vi "GetMTSUMData.vi"(10 "RCNO":string="A150100736") -> (0 "bin4":i32, 1 "bin3":i32, 2 "bin2":i32, 3 "bin1":i32, 4 "Program":string, 5 "input":i32, 6 "EndDate":string, 7 "StartDate":string, 8 "Yield":dbl)   [LabVIEW 2012]
uses:
  <vilib>/addons/database/Auxilliary.llb/DB Tools Cursor Type.ctl
  <vilib>/addons/database/Connection.llb/DB Tools Open Connec (Path).vi
  <vilib>/addons/database/Connection.llb/Conn Execute.vi
  <vilib>/addons/database/Recordset.llb/Rec Fetch String Data (R).vi
  <vilib>/addons/database/Recordset.llb/Rec Fetch Integer Data (R).vi
  <vilib>/addons/database/Recordset.llb/Rec Destroy - Connection.vi
  <vilib>/addons/database/NI_Database_API.lvlib
panel:
  out "error out":errorcluster
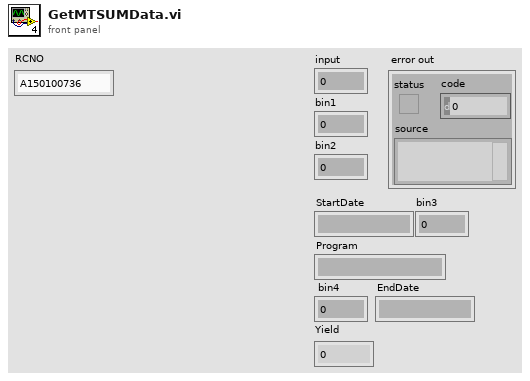
[diagram p1: front panel]
types:
  T1 = typedef "NI_Database_API.lvlib/DB Tools Cursor Type.ctl" = enum16{"forward-only", "keyset", "dynamic", "static"}
  T2 = typedef "NI_Database_API.lvlib/Conn ObjectReference.ctl" = refnum<k1>
  T3 = typedef "NI_Database_API.lvlib/Rec ObjectReference.ctl" = refnum<k1>
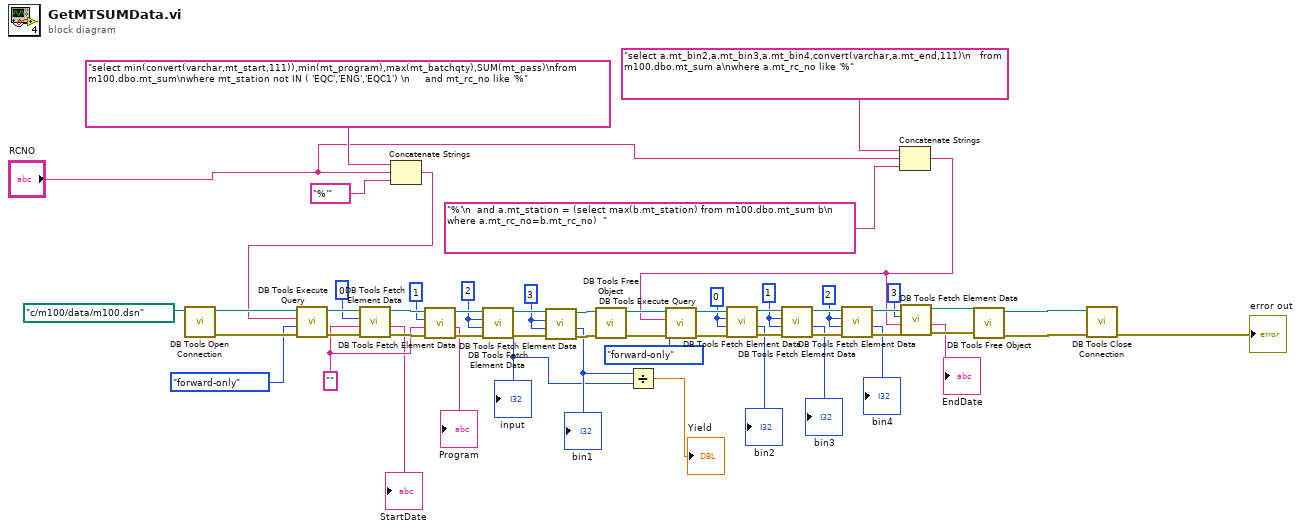
[diagram p0: block diagram]
diagram:
  w23 = 2
  w24 = 1
  w25 = 0
  w38 = 3
  w39 = 2
  w42 = ""
  n1 = call-poly <vilib>:"DB Tools Open Connection.vi"("connection information"=path "c:/m100/data/m100.dsn") -> ("error out"=w52:errorcluster, "connection reference"=w54:T2)  [unwired: 7 in]
  n2 = Concatenate Strings("select min(convert(varchar,mt_start,111)),min(mt_program),max(mt_batchqty),SUM(mt_pass)\nfrom m100.dbo.mt_sum\nwhere mt_station not IN ( 'EQC','ENG','EQC1') \n     and mt_rc_no like '%", "RCNO", "%'" ("string")) -> (w16:string)
  n3 = call-poly <vilib>:"DB Tools Execute Query.vi"("error in (no error)"=w52, "cursor type"=DB_Tools_Cursor_Type."forward-only", "SQL query"=w16, "connection reference"=w54) -> ("error out"=w51:errorcluster, "recordset reference"=w53:T3)  [unwired: 4 in]
  n4 = call-poly <vilib>:"DB Tools Fetch Element Data.vi"("error in (no error)"=w51, "type"=w42, "column index"=0, "recordset reference"=w53) -> ("error out"=w48:errorcluster, "data"=→"StartDate":string, "recordset reference out"=w47:T3)  [unwired: 3 in]
  n5 = call-poly <vilib>:"DB Tools Fetch Element Data.vi"("error in (no error)"=w48, "type"=w42, "column index"=1, "recordset reference"=w47) -> ("error out"=w43:errorcluster, "data"=→"Program":string, "recordset reference out"=w44:T3)  [unwired: 3 in]
  n6 = call-poly <vilib>:"DB Tools Fetch Element Data.vi"("error in (no error)"=w43, "type"=w39, "column index"=w39, "recordset reference"=w44) -> ("error out"=w46:errorcluster, "data"=w17:i32, "recordset reference out"=w45:T3)  [unwired: 3 in]
  "input" <- w17
  n7 = call-poly <vilib>:"DB Tools Fetch Element Data.vi"("error in (no error)"=w46, "type"=w38, "column index"=w38, "recordset reference"=w45) -> ("error out"=w34:errorcluster, "data"=w18:i32, "recordset reference out"=w35:T3)  [unwired: 3 in]
  "bin1" <- w18
  n8 = call-poly <vilib>:"DB Tools Free Object.vi"("error in (no error)"=w34, "recordset reference"=w35) -> ("error out"=w32:errorcluster, "connection reference"=w33:T2)  [unwired: 8 in]
  n9 = Divide(x=w18, y=w17) -> (x/y=→"Yield":dbl)
  n10 = Concatenate Strings("select a.mt_bin2,a.mt_bin3,a.mt_bin4,convert(varchar,a.mt_end,111)\n   from m100.dbo.mt_sum a\nwhere a.mt_rc_no like '%" ("SQL query"), "RCNO", "%'\n  and a.mt_station = (select max(b.mt_station) from m100.dbo.mt_sum b\n                      where a.mt_rc_no=b.mt_rc_no)  " ("SQL query")) -> (w4:string)
  n11 = call-poly <vilib>:"DB Tools Execute Query.vi"("error in (no error)"=w32, "cursor type"=DB_Tools_Cursor_Type."forward-only", "SQL query"=w4, "connection reference"=w33) -> ("error out"=w26:errorcluster, "recordset reference"=w27:T3)  [unwired: 4 in]
  n12 = call-poly <vilib>:"DB Tools Fetch Element Data.vi"("error in (no error)"=w26, "type"=w25, "column index"=w25, "recordset reference"=w27) -> ("error out"=w31:errorcluster, "data"=→"bin2":i32, "recordset reference out"=w30:T3)  [unwired: 3 in]
  n13 = call-poly <vilib>:"DB Tools Fetch Element Data.vi"("error in (no error)"=w31, "type"=w24, "column index"=w24, "recordset reference"=w30) -> ("error out"=w29:errorcluster, "data"=→"bin3":i32, "recordset reference out"=w28:T3)  [unwired: 3 in]
  n14 = call-poly <vilib>:"DB Tools Fetch Element Data.vi"("error in (no error)"=w29, "type"=w23, "column index"=w23, "recordset reference"=w28) -> ("error out"=w9:errorcluster, "data"=→"bin4":i32, "recordset reference out"=w7:T3)  [unwired: 3 in]
  n15 = call-poly <vilib>:"DB Tools Fetch Element Data.vi"("error in (no error)"=w9, "type"=w4, "column index"=3, "recordset reference"=w7) -> ("error out"=w5:errorcluster, "data"=→"EndDate":string, "recordset reference out"=w6:T3)  [unwired: 3 in]
  n16 = call-poly <vilib>:"DB Tools Free Object.vi"("error in (no error)"=w5, "recordset reference"=w6) -> ("error out"=w21:errorcluster, "connection reference"=w22:T2)  [unwired: 8 in]
  n17 = call <vilib>:"DB Tools Close Connection.vi"("error in (no error)"=w21, "connection reference"=w22) -> ("error out"=→"error out":errorcluster)  [unwired: 5 in]
